vi "PROXY_translate_tray_menu.vi"(6 "NotifyIcon reference in":refnum<k24>, 8 "error_in":errorcluster) -> (0 "error_out":errorcluster)   [LabVIEW 2020]
uses:
  System.Windows.Forms
  _misc/NotifyIcon/TypeDefs/NotifyIcon Event Registration Actions.ctl
  _misc/NotifyIcon/TypeDefs/NotifyIcon Events.ctl
  _misc/AULocalize/SubVIs/Get Localized Phrase Compact Interface 2D.vi
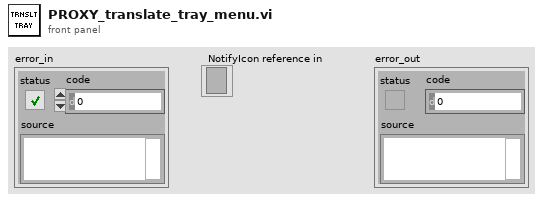
[diagram p1: front panel]
types:
  T1 = typedef "NotifyIcon Events.ctl" = enum16{"BalloonTipClicked", "BalloonTipClosed", "BalloonTipShown", "Click", "Disposed", "DoubleClick", "MouseClick", "MouseDoubleClick", "MouseDown", "MouseMove", "MouseUp", "MenuItemClick", "MenuItemSelect"}
  T2 = typedef "NotifyIcon Event Registration Actions.ctl" = enum16{"Initial Event Registration", "Add to Event Registration", "Destroy Events and Re-register"}
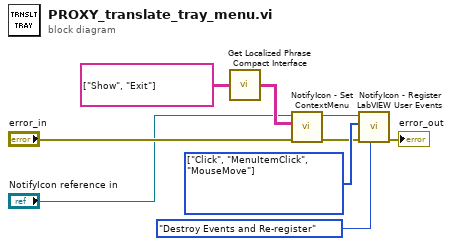
[diagram p0: block diagram]
diagram:
  w8 = T1[] [enum."Click", enum."MenuItemClick", enum."MouseMove"] items=["BalloonTipClicked", "BalloonTipClosed", "BalloonTipShown", "Click", "Disposed", "DoubleClick", "MouseClick", "MouseDoubleClick", "MouseDown", "MouseMove", "MouseUp", "MenuItemClick", "MenuItemSelect"] ("Events to register")
  n1 = call-poly "Get Localized Phrase Compact Interface.vi"("Key"=string[][] [["Show"], ["Exit"]] ("Context Menu (optional)")) -> ("Translated Phrase"=w5:string[][])
  n2 = call "NotifyIcon - Set ContextMenu.vi"("error in"="error_in", "Context Menu"=w5, "NotifyIcon reference in"="NotifyIcon reference in") -> ("error out"=w7:errorcluster, "NotifyIcon reference out"=w9:refnum<k24>)  [unwired: 7 in]
  n3 = call "NotifyIcon - Register LabVIEW User Events.vi"("Action"=NotifyIcon_Event_Registration_Actions."Destroy Events and Re-register", "error in"=w7, "Events to register"=w8, "NotifyIcon reference in"=w9) -> ("error out"=→"error_out":errorcluster)  [unwired: 5 in, 2 out]
